vi "Configure.vi"(8 "error in (no error)":errorcluster, 10 "ID":string, 11 "SimGauge in":refnum<class "SimGauge.lvclass">) -> (0 "error out":errorcluster, 3 "SimGauge out":refnum<class "SimGauge.lvclass">)   [LabVIEW 2016, in "SimGauge.lvlib" / "SimGauge.lvclass"]
uses:
  SimGauge.lvclass
  SimGauge.lvclass/SimGauge.ctl
  <vilib>/Utility/config.llb/Read Key (Double).vi
  <vilib>/Utility/config.llb/NI_LVConfig.lvlib
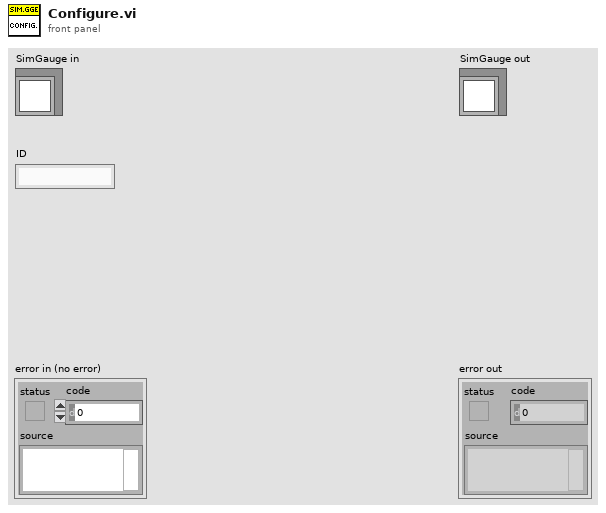
[diagram p1: front panel]
types:
  T1 = typedef "NI_LVConfig.lvlib/Config Data RefNum.ctl" = refnum<k1>
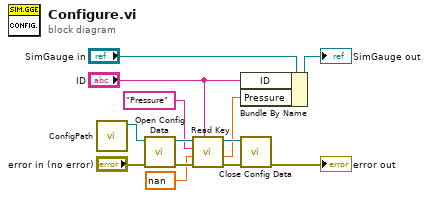
[diagram p0: block diagram]
diagram:
  n1 = call "ConfigPath.vi"() -> ("ConfigPath"=w12:path)  [unwired: 11 in]
  n2 = call <vilib>:"Open Config Data.vi"("error in (no error)"="error in (no error)", "configuration file path"=w12) -> ("error out"=w10:errorcluster, "refnum"=w11:T1)  [unwired: 7 in, 1 out]
  n3 = call-poly <vilib>:"Read Key.vi"("section"="ID", "error in (no error)"=w10, "default value"=nan, "key"="Pressure", "refnum"=w11) -> ("error out"=w7:errorcluster, "value"=w5:dbl, "refnum out"=w6:T1)  [unwired: 3 in, 1 out]
  n4 = Bundle By Name(cluster="SimGauge in", "ID"="ID", "Pressure"=w5) -> (→"SimGauge out":refnum<class "SimGauge.lvclass">)
  n5 = call <vilib>:"Close Config Data.vi"("error in (no error)"=w7, "refnum"=w6) -> ("error out"=→"error out":errorcluster)  [unwired: 8 in, 1 out]
